vi "AM Rx.vi"() -> ()   [LabVIEW 2011]
doc: "This example <B>requires the Modulation Toolkit</B>.\n\nContinuously acquires FM radio, demodulates and plays the result back through your PC sound card. The acquired signal is resampled to a rate appropriate for the sound card. Only the mono component of the signal is played back-additional signal processing would be required to recover both audio channels to enable stereo playback.\n\nOn the LabVIEW diagram, two separate loops are used to enable multi-rate processing. Multi-rate processing enables the section of the VI that handles the acquisition to run at a different rate than the section of code that handles demodulation. The top loop handles the acquisition, calling the NI-USRP driver to request incoming signal samples. The bottom loop processes the acquired signal, performing the resampling, demodulation, display and interface with the sound card. A queue is used to transfer signal samples from the top loop to the bottom loop."
uses:
  <vilib>/sound2/lvsound2.llb/Sound Data Format.ctl
  <vilib>/sound2/lvsound2.llb/Sampling Mode.ctl
  <vilib>/sound2/lvsound2.llb/Sound Output Write (DBL Single).vi
  <instrlib>/niUSRP/niUSRP Fetch Rx Data (CDB Cluster).vi
  <vilib>/addons/Modulation/Analog/MT Demodulate AM (DSB).vi
  <vilib>/measure/maresamp.llb/Resample Waveform (single shot).vi
  <vilib>/measure/NI_MAPro.lvlib
  <vilib>/addons/Modulation/niAMT.lvlib
panel:
  out "Acq & Proc\nLoop Status":bool
  out "Gain [dB] (actual)":dbl=20.0 format="%#.6p"
  out "Carrier Frequency \n[Hz] (actual)":dbl=90499999.99533428 format="%#.6p"
  out "IQ Sampling\nRate [s/sec] (actual)":dbl=200000.0 format="%#.6p"
  in  "Active Antenna":string(combo)="RX1"
  in  "Gain [dB]":dbl=20.0 format="%#.6p"
  in  "Carrier\nFrequency [Hz]":dbl=90500000.0 format="%#.6p"
  in  "IQ Sampling\nRate [s/sec]":dbl=200000.0 format="%#.6p"
  in  "device names":refnum<k15>="192.168.10.3"
  in  "stop":bool
  in  "Tab Control":enum32{"FM Demod Display", "Parameters"}(tab)
  out "AM Demodulated":waveform(dbl)(graph)
  out "carrier amplitude":dbl format="%.2f"
  in  "Modulation Index":dbl=30000.0 format="%.2p"
  out "Samples per\nFrame":i64=200000
  in  "Seconds\nper Frame":dbl=1.0
  in  "sound format":T1={"sample rate (S/s)"=44100.0, "number of channels"=2, "bits per sample"=16}
  in  "Sound Card ID":u32
  in  "FIR filter specifications\nfor Resampling":T2={"alias rejection (dB)"=40.0, "normalized bandwidth"=0.3} {"normalized bandwidth" format="%.4f"; "alias rejection (dB)" format="%.2f"}
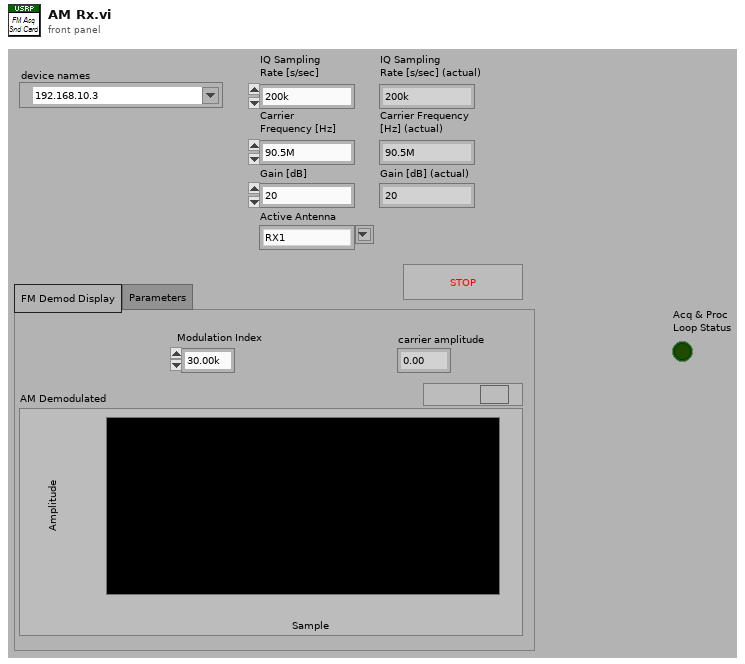
[diagram p1: front panel]
types:
  T1 = typedef "Sound Data Format.ctl" = cluster{"sample rate (S/s)":dbl, "number of channels":i32, "bits per sample":i32}
  T2 = cluster{"alias rejection (dB)":dbl, "normalized bandwidth":dbl}
  T3 = typedef "Sampling Mode.ctl" = i32
  T4 = typedef "Sound Output Task ID.ctl" = u32
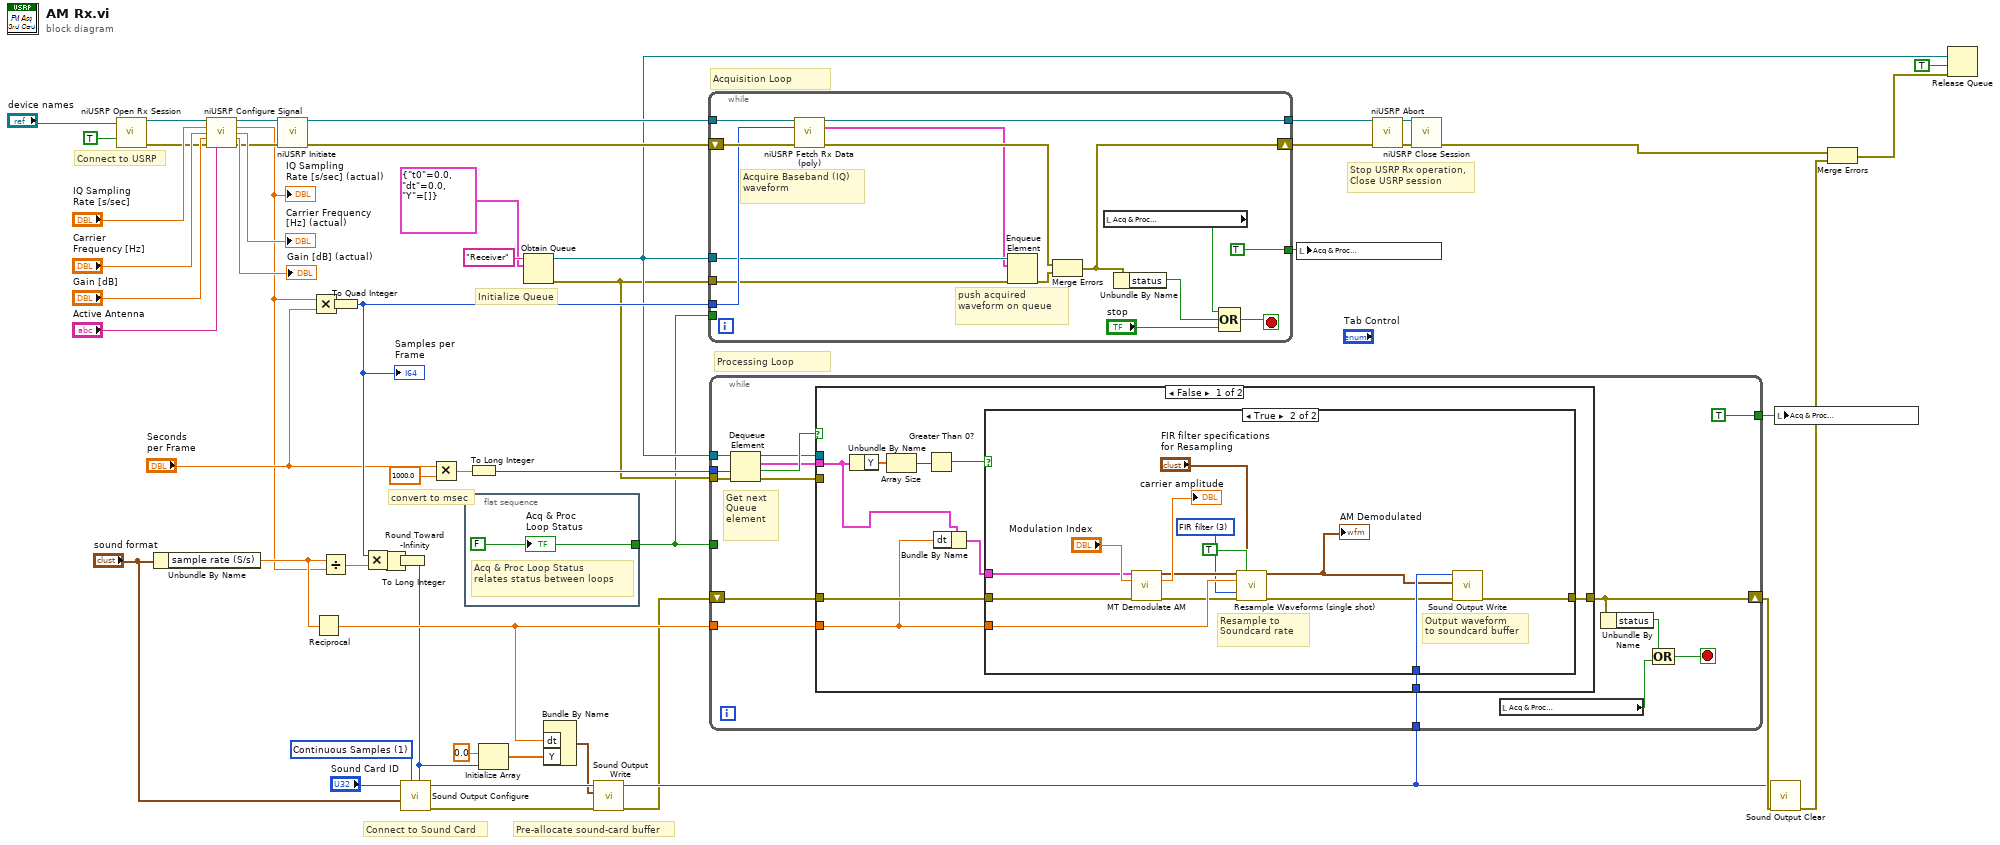
[diagram p0: block diagram]
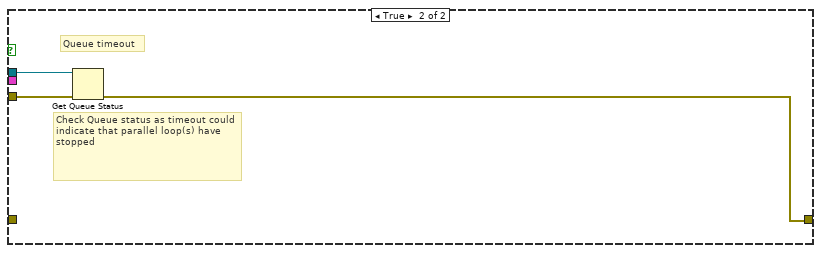
[diagram p3: hidden frame]
diagram:
  w53 = T3 1 items=["Finite Samples", "Continuous Samples"] ("sample mode")
  # "convert to msec"
  # "Initialize Queue"
  # "Stop USRP Rx operation,\nClose USRP session"
  # "Processing Loop"
  # "Acquisition Loop"
  # "Connect to USRP"
  # "Pre-allocate sound-card buffer"
  # "Connect to Sound Card"
  n1 = call <instrlib>:"niUSRP Open Rx Session.vi"("device names"="device names", "reset"=TRUE) -> ("session handle out"=w9:refnum<k15>, "error out"=w8:errorcluster)  [unwired: 12 in]
  n2 = Unbundle By Name("sound format") -> ("sample rate (S/s)"=w42:dbl)
  n3 = call <instrlib>:"niUSRP Configure Signal.vi"("session handle"=w9, "IQ rate"="IQ Sampling\nRate [s/sec]", "carrier frequency"="Carrier\nFrequency [Hz]", "gain"="Gain [dB]", "error in (no error)"=w8, "active antenna"="Active Antenna") -> ("session handle out"=w6:refnum<k15>, "coerced IQ rate"=w5:dbl, "coerced carrier frequency"=→"Carrier Frequency \n[Hz] (actual)":dbl, "coerced gain"=→"Gain [dB] (actual)":dbl, "error out"=w7:errorcluster)  [unwired: 5 in]
  "IQ Sampling\nRate [s/sec] (actual)" <- w5
  n4 = call <instrlib>:"niUSRP Initiate.vi"("session handle"=w6, "error in (no error)"=w7) -> ("session handle out"=w40:refnum<k15>, "error out"=w39:errorcluster)  [unwired: 12 in]
  n5 = Multiply(x=w5, y="Seconds\nper Frame") -> (x*y=w34:dbl)
  n6 = Reciprocal(x=w42) -> (1/x=w43:dbl)
  n7 = Divide(x=w42, y=w5) -> (x/y=w45:dbl)
  n8 = To Quad Integer(1:w34) -> (0:w33:i64)
  "Samples per\nFrame" <- w33
  n9 = Multiply(x=w33, y=w45) -> (x*y=w47:dbl)
  n10 = Round Toward -Infinity(1:w47) -> (0:w46:dbl)
  n11 = To Long Integer(number=w46) -> (32bit integer=w41:i32)
  n12 = call <vilib>:"Sound Output Configure.vi"("number of samples/ch"=w41, "sample mode"=w53, "sound format"="sound format", "device ID"="Sound Card ID") -> ("error out"=w50:errorcluster, "task ID"=w49:T4)  [unwired: 6 in]
  n13 = Multiply(x="Seconds\nper Frame", y=1000.0) -> (x*y=w29:dbl)
  n14 = flat-sequence {
    tunnel: [w54] -> w1
    frame #0 {
      w54 = FALSE ("Acq & Proc\nLoop Status")
      # "Acq & Proc Loop Status \nrelates status between loops"
      "Acq & Proc\nLoop Status" <- w54
    }
  }
  n15 = To Long Integer(number=w29) -> (32bit integer=w28:i32)
  n16 = Initialize Array(0.0 ("element"), w41) -> (w44:dbl[])
  n17 = Obtain Queue(name (unnamed)="Receiver", element data type=cluster{"t0":dbl, "dt":dbl, "Y":cdb[]} {"t0"=0.0, "dt"=0.0, "Y"=[]} ("data")) -> (queue out=w20:refnum<queue>, error out=w17:errorcluster)  [unwired: 3 in, 1 out]
  n18 = Bundle By Name("dt"=w43, "Y"=w44) -> (w27:waveform(dbl))  [unwired: 1 in]
  n19 = call-poly <vilib>:"Sound Output Write.vi"("error in (no error)"=w50, "data"=w27, "task ID"=w49) -> ("error out"=w24:errorcluster, "task ID out"=w25:T4)  [unwired: 7 in]
  n20 = while {
    tunnel: w40 -> [w69]
    tunnel: [w68] -> w38
    tunnel: w33 -> [w66]
    tunnel: w20 -> [w63]
    shift-right: [w60] -> w37
    shift-left: w39 -> [w67]
    tunnel: w17 -> [w61]
    tunnel: [TRUE ("Acquisition & Processing\nLoop Status")] -> w4
    tunnel: w1 -> [_]
    stop <- w65 stop-if-true
    # "push acquired waveform on queue"
    # "Acquire Baseband (IQ) waveform"
    n21 = call-poly <instrlib>:"niUSRP Fetch Rx Data (poly).vi"("session handle"=w69, "number of samples"=w66, "error in (no error)"=w67) -> ("session handle out"=w68:refnum<k15>, "data"=w55:cluster{"t0":dbl, "dt":dbl, "Y":cdb[]}, "error out"=w59:errorcluster)  [unwired: 9 in, 1 out]
    n22 = Enqueue Element(queue=w63, element=w55, error in (no error)=w61) -> (error out=w62:errorcluster)  [unwired: 1 in, 2 out]
    n23 = Merge Errors(w59, w62) -> (w60:errorcluster)
    n24 = local read "Acq & Proc\nLoop Status"() -> (w56:bool)
    n25 = Unbundle By Name(w60) -> ("status"=w64:bool)
    n26 = Compound Arithmetic op=OR(w56, w64, "stop") -> (w65:bool)
  }
  n27 = while {
    tunnel: w43 -> [w84]
    tunnel: w20 -> [w76]
    tunnel: w28 -> [w83]
    shift-right: [w78] -> w26
    shift-left: w24 -> [w80]
    tunnel: w25 -> [w79]
    tunnel: w17 -> [w75]
    tunnel: [TRUE ("Acquisition & Processing\nLoop Status")] -> w3
    tunnel: w1 -> [_]
    stop <- w72 stop-if-true
    # "Get next Queue element"
    n28 = Dequeue Element(queue=w76, timeout in ms (-1)=w83, error in (no error)=w75) -> (queue out=w73:refnum<queue>, element=w81:cluster{"t0":dbl, "dt":dbl, "Y":cdb[]}, timed out?=w82:bool, error out=w74:errorcluster)
    n29 = case shown="False" w82 {
      tunnel: w84 -> [w86 _]
      tunnel: w81 -> [w87 _]
      tunnel: w80 -> [w91 _]
      tunnel: [w90 w109] -> w78
      tunnel: w79 -> [w89 _]
      tunnel: w74 -> [_ w111]
      tunnel: w73 -> [_ w110]
      frame False {
        n30 = Unbundle By Name(w87) -> ("Y"=w93:cdb[])
        n31 = Array Size(array=w93) -> (size(s)=w92:i32)
        n32 = Greater Than 0?(x=w92) -> (x > 0?=w88:bool)
        n33 = Bundle By Name(cluster=w87, "dt"=w86) -> (w85:cluster{"t0":dbl, "dt":dbl, "Y":cdb[]})
        n34 = case shown="True" w88 {
          tunnel: w86 -> [_ w108]
          tunnel: w85 -> [_ w101]
          tunnel: w91 -> [w94 w97]
          tunnel: [w94 w100] -> w90
          tunnel: w89 -> [_ w98]
          frame False {
            # "Empty buffer or stop button pressed, don't process"
          }
          frame True {
            w103 = u16 3 items=["coerce", "linear", "spline", "FIR filter"] ("interpolation mode")
            # "Output waveform \nto soundcard buffer"
            # "Resample to Soundcard rate"
            n35 = call-poly <vilib>:"MT Demodulate AM.vi"("AM modulated waveform"=w101, "modulation index"="Modulation Index", "error in (no error)"=w97) -> ("AM demodulated waveform"=w104:waveform(dbl), "carrier amplitude"=→"carrier amplitude":dbl, "error out"=w105:errorcluster)  [unwired: 10 in]
            n36 = call-poly <vilib>:"Resample Waveforms (single shot).vi"("waveform in"=w104, "open interval? (F)"=TRUE, "dt"=w108, "interpolation mode"=w103, "error in (no error)"=w105, "FIR filter specifications"="FIR filter specifications\nfor Resampling") -> ("resampled waveform out"=w95:waveform(dbl), "error out"=w96:errorcluster)  [unwired: 6 in, 2 out]
            "AM Demodulated" <- w95
            n37 = call-poly <vilib>:"Sound Output Write.vi"("error in (no error)"=w96, "data"=w95, "task ID"=w98) -> ("error out"=w100:errorcluster)  [unwired: 7 in, 1 out]
          }
        }
      }
      frame True {
        # "Queue timeout"
        # "Check Queue status as timeout could indicate that parallel loop(s) have stopped"
        n38 = Get Queue Status(queue=w110, error in (no error)=w111) -> (error out=w109:errorcluster)  [unwired: 1 in, 7 out]
      }
    }
    n39 = local read "Acq & Proc\nLoop Status"() -> (w70:bool)
    n40 = Unbundle By Name(w78) -> ("status"=w77:bool)
    n41 = Compound Arithmetic op=OR(w77, w70) -> (w72:bool)
  }
  n42 = local write "Acq & Proc\nLoop Status"(w4) -> ()
  n43 = call <instrlib>:"niUSRP Abort.vi"("session handle"=w38, "error in (no error)"=w37) -> ("session handle out"=w36:refnum<k15>, "error out"=w35:errorcluster)  [unwired: 12 in]
  n44 = call <instrlib>:"niUSRP Close Session.vi"("session handle"=w36, "error in (no error)"=w35) -> ("error out"=w23:errorcluster)  [unwired: 13 in]
  n45 = call <vilib>:"Sound Output Clear.vi"("error in (no error)"=w26, "task ID"=w25) -> ("error out"=w22:errorcluster)  [unwired: 9 in]
  n46 = local write "Acq & Proc\nLoop Status"(w3) -> ()
  n47 = Merge Errors(w23, w22) -> (w21:errorcluster)
  n48 = Release Queue(queue=w20, force destroy? (F)=TRUE, error in (no error)=w21) -> ()  [unwired: 3 out]
